vi "ErrorCalculate.vi"(5 "RingdownParameters":T1, 6 "error in":errorcluster, 7 "input_data":dbl[](array[numeric]), 8 "num_modes":dbl, 9 "time":dbl[](array[numeric]), 10 "nnfit":dbl, 11 "dft":dbl) -> (0 "input_data":dbl[](array[numeric]), 1 "null_input":dbl[](array[numeric]), 2 "error_sig":dbl[](array[numeric]), 3 "prony_estimate":dbl[](array[numeric]), 4 "error out":errorcluster)   [LabVIEW 2017, in "Visualization.lvlib" / "VisualizeAppRingdown.lvclass"]
uses:
  VisualizeAppRingdown.lvclass
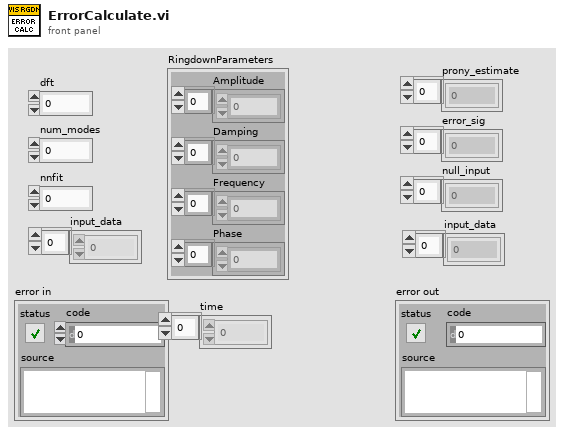
[diagram p1: front panel]
types:
  T1 = cluster{"Amplitude":dbl[], "Damping":dbl[], "Frequency":dbl[], "Phase":dbl[]}
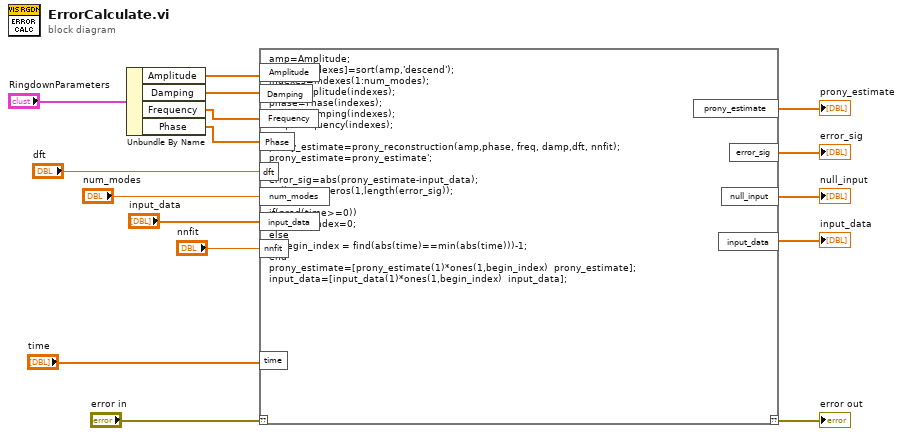
[diagram p0: block diagram]
diagram:
  n1 = Unbundle By Name("RingdownParameters") -> ("Amplitude"=w15:dbl[], "Damping"=w14:dbl[], "Frequency"=w13:dbl[], "Phase"=w12:dbl[])
  n2 = script code="amp=Amplitude;\n[values indexes]=sort(amp,'descend');\nindexes=indexes(1:num_modes);\namp=Amplitude(indexes);\nphase=Phase(indexes);\ndamp=Damping(indexes);\nfreq=Frequency(indexes);\n\nprony_estimate=prony_reconstruction(amp,phase, freq, damp,dft, nnfit);\nprony_estimate=prony_estimate';\n\nerror_sig=abs(prony_estimate-input_data);\nnull_input=zeros(1,length(error_sig));\n\nif(prod(time>=0))\n    begin_index=0;\nelse\n    begin_index = find(abs(time)==min(abs(time)))-1;\nend\nprony_estimate=[prony_estimate(1)*ones(1,begin_index)  prony_estimate];\ninput_data=[input_data(1)*ones(1,begin_index)  input_data];"("??"="error in", "dft"="dft", "num_modes"="num_modes", "input_data"="input_data", "nnfit"="nnfit", "Amplitude"=w15, "Damping"=w14, "Frequency"=w13, "Phase"=w12, "time"="time") -> ("??"=→"error out":errorcluster, "prony_estimate"=→"prony_estimate":dbl[], "error_sig"=→"error_sig":dbl[], "null_input"=→"null_input":dbl[], "input_data"=→"input_data":dbl[])
